vi "HV_drive.vi"(3 "Stop subVI Refnum":refnum<vi>, 4 "HV level Refnum":refnum<vi>, 5 "HV parameters":T1={"Final value"=-1000, "Number of steps"=10, "Time/step"=500, "Output Off Behavior"=0, "VISA resource name"="GPIB0::25::INSTR"} {"Output Off Behavior" items=["Normal", "High Impedance", "Zero", "Guard"]; "Time/step" min=100 max=2000 step=100; "Final value" min=-1100 max=0 step=10; "Number of steps" min=10 max=20 step=10}) -> (0 "error out":errorcluster, 2 "HV level (last value)":dbl(slide) scale=0.0..-1000.0)   [LabVIEW 2015, in "VIPM2.lvlib"]
uses:
  VIPM2.lvlib
  dr_Keithley 24XX/Keithley 24XX.lvlib
panel:
  # "Driver for the High Voltage Power Supply"
  # "Executa rampa de pujada o rampa de baixada"
  # "V"
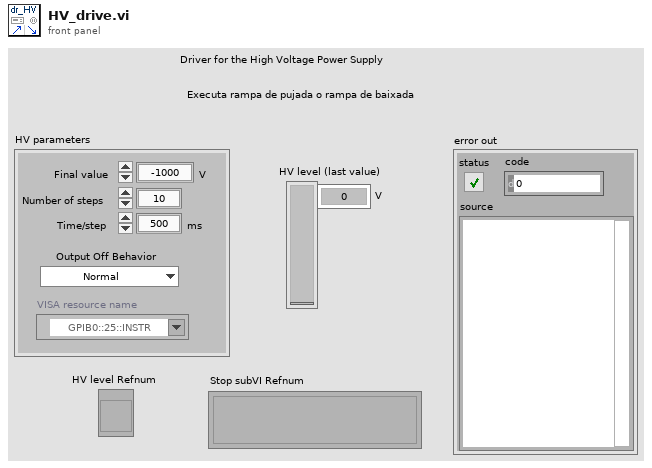
[diagram p1: front panel]
types:
  T1 = cluster{"Final value":i16, "Number of steps":u8, "Time/step":u16, "Output Off Behavior":u16, "VISA resource name":refnum<visa-resource-name>}
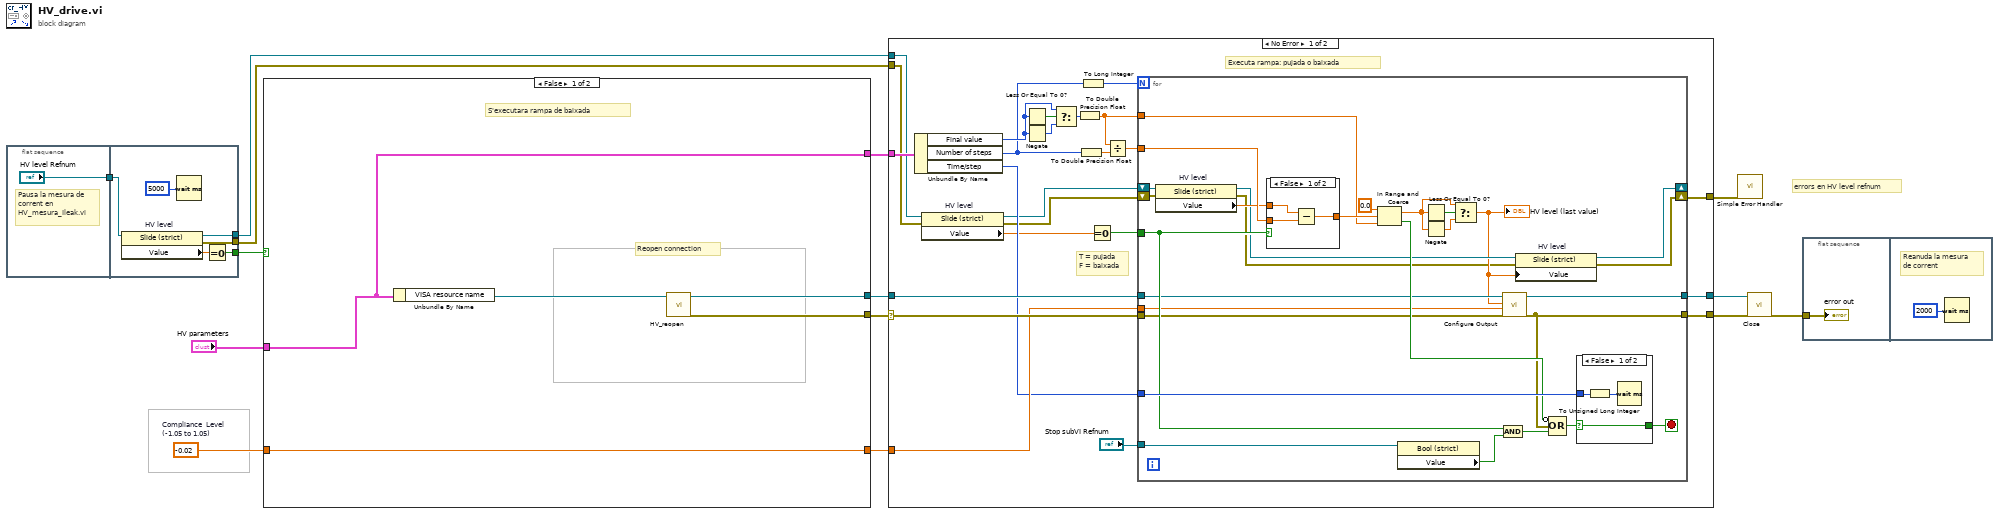
[diagram p0: block diagram]
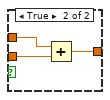
[diagram p3: hidden frame]
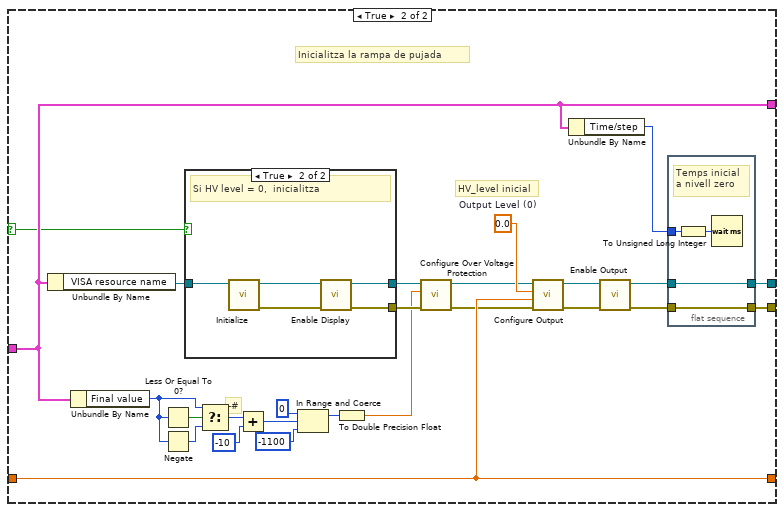
[diagram p5: hidden frame]
diagram:
  w12 = -0.02  # Compliance  Level (-1.05 to 1.05)
  # "errors en HV level refnum"
  n1 = flat-sequence {
    tunnel: ["HV level Refnum"] -> w7
    tunnel: [w21] -> w13
    tunnel: w7 -> [w19]
    tunnel: [w17] -> w6
    tunnel: [w16] -> w5
    frame #0 {
      # "Pausa la mesura de\ncorrent en\nHV_mesura_Ileak.vi"
    }
    frame #1 {
      n2 = property on="HV level" class="Slide (strict)"(reference=w19) -> (reference out=w17:refnum<vi>, error out=w16:errorcluster, "Value"=w18:dbl)  [unwired: 1 in]
      n3 = Wait (ms)(milliseconds to wait=u32 5000) -> ()  [unwired: 1 out]
      n4 = Equal To 0?(x=w18) -> (x = 0?=w21:bool)
    }
  }
  n5 = case shown="False" w13 {
    selector: w13 -> [_ w27]
    tunnel: "HV parameters" -> [w25 w40]
    tunnel: w12 -> [w26 w34]
    tunnel: [w24 w41] -> w9
    tunnel: [w23 w42] -> w10
    tunnel: [w26 w34] -> w8
    tunnel: [w25 w40] -> w11
    frame False {
      # "Reopen connection"
      # "S'executara rampa de baixada"
      n6 = Unbundle By Name(w25) -> ("VISA resource name"=w22:refnum<visa-resource-name>)
      n7 = call "HV_reopen.vi"("VISA resource name"=w22) -> ("error out"=w23:errorcluster, "VISA resource name out"=w24:refnum<visa-resource-name>)  [unwired: 9 in]
    }
    frame True {
      w33 = 0.0  # Output Level (0)
      # "HV_level inicial"
      # "Inicialitza la rampa de pujada"
      # "-#"
      n8 = Unbundle By Name(w40) -> ("VISA resource name"=w52:refnum<visa-resource-name>)
      n9 = Unbundle By Name(w40) -> ("Final value"=w50:i16)
      n10 = Less Or Equal To 0?(x=w50) -> (x <= 0?=w51:bool)
      n11 = Negate(x=w50) -> (-x=w49:i16)
      n12 = case shown="True" w27 {
        tunnel: [w53 w58] -> w29
        tunnel: [_ w57] -> w30
        tunnel: w52 -> [w53 w54]
        frame False {
        }
        frame True {
          # "Si HV level = 0,  inicialitza"
          n13 = call "Initialize.vi"("VISA resource name"=w54) -> ("error out"=w56:errorcluster, "VISA resource name out"=w55:refnum<visa-resource-name>)  [unwired: 9 in]
          n14 = call "Enable Display.vi"("error in (no error)"=w56, "VISA resource name"=w55) -> ("error out"=w57:errorcluster, "VISA resource name out"=w58:refnum<visa-resource-name>)  [unwired: 8 in]
        }
      }
      n15 = Select(t=w50, s=w51, f=w49) -> (s? t:f=w48:i16)
      n16 = Add(x=w48, y=i16 -10) -> (x+y=w46:i16)
      n17 = In Range and Coerce(upper limit=i16 0, x=w46, lower limit=i16 -1100) -> (coerced(x)=w43:i16)  [unwired: 1 out]
      n18 = To Double Precision Float(number=w43) -> (double precision float=w28:dbl)
      n19 = call "Configure Over Voltage Protection.vi"("error in (no error)"=w30, "Voltage Limit (0.0 V)"=w28, "VISA resource name"=w29) -> ("error out"=w32:errorcluster, "VISA resource name out"=w31:refnum<visa-resource-name>)  [unwired: 7 in]
      n20 = call "Configure Output.vi"("error in (no error)"=w32, "Compliance  Level (0.1)"=w34, "Output Level (0)"=w33, "VISA resource name"=w31) -> ("error out"=w36:errorcluster, "VISA resource name out"=w35:refnum<visa-resource-name>)  [unwired: 6 in]
      n21 = Unbundle By Name(w40) -> ("Time/step"=w39:u16)
      n22 = call "Enable Output.vi"("error in (no error)"=w36, "VISA resource name"=w35) -> ("error out"=w38:errorcluster, "VISA resource name out"=w37:refnum<visa-resource-name>)  [unwired: 8 in]
      n23 = flat-sequence {
        tunnel: w38 -> [w62]
        tunnel: [w62] -> w42
        tunnel: w37 -> [w61]
        tunnel: [w61] -> w41
        tunnel: w39 -> [w60]
        frame #0 {
          # "Temps inicial\na nivell zero"
          n24 = To Unsigned Long Integer(number=w60) -> (unsigned 32bit integer=w59:u32)
          n25 = Wait (ms)(milliseconds to wait=w59) -> ()  [unwired: 1 out]
        }
      }
    }
  }
  n26 = case shown="No Error" w10 {
    selector: w10 -> [w84 w126]
    tunnel: w11 -> [w86 _]
    tunnel: w9 -> [w85 w127]
    tunnel: w8 -> [w83 _]
    tunnel: [w79 w127] -> w2
    tunnel: [w78 w126] -> w3
    tunnel: w6 -> [w69 _]
    tunnel: w5 -> [w65 w125]
    tunnel: [w64 w125] -> w4
    frame No Error {
      # "Executa rampa: pujada o baixada"
      # "T = pujada\nF = baixada"
      n27 = Unbundle By Name(w86) -> ("Final value"=w75:i16, "Number of steps"=w70:u8, "Time/step"=w80:u16)
      n28 = property on="HV level" class="Slide (strict)"(reference=w69, error in=w65) -> (reference out=w67:refnum<vi>, error out=w66:errorcluster, "Value"=w68:dbl)
      n29 = Less Or Equal To 0?(x=w75) -> (x <= 0?=w76:bool)
      n30 = Negate(x=w75) -> (-x=w77:i16)
      n31 = Select(t=w75, s=w76, f=w77) -> (s? t:f=w74:i16)
      n32 = To Double Precision Float(number=w74) -> (double precision float=w73:dbl)
      n33 = To Double Precision Float(number=w70) -> (double precision float=w72:dbl)
      n34 = To Long Integer(number=w70) -> (32bit integer=w71:i32)
      n35 = Equal To 0?(x=w68) -> (x = 0?=w81:bool)
      n36 = Divide(x=w73, y=w72) -> (x/y=w82:dbl)
      n37 = for {
        N: w71 -> [_]
        tunnel: w85 -> [w98]
        tunnel: w84 -> [w99]
        tunnel: w83 -> [w97]
        tunnel: w82 -> [w114]
        tunnel: w81 -> [w111]
        tunnel: [w100] -> w79
        tunnel: [w101] -> w78
        tunnel: w80 -> [w113]
        tunnel: w73 -> [w104]
        shift-right: [w92] -> _
        shift-left: w67 -> [w96]
        shift-right: [w89] -> w64
        shift-left: w66 -> [w90]
        tunnel: "Stop subVI Refnum" -> [w88]
        stop <- w102 stop-if-true
        n38 = property on="HV level" class="Slide (strict)"(reference=w96, error in=w90) -> (reference out=w94:refnum<vi>, error out=w91:errorcluster, "Value"=w95:dbl)
        n39 = case shown="False" w111 {
          tunnel: w114 -> [w121 w122]
          tunnel: [w120 w124] -> w110
          tunnel: w95 -> [w119 w123]
          frame False {
            n40 = Subtract(x=w119, y=w121) -> (x-y=w120:dbl)
          }
          frame True {
            n41 = Add(x=w123, y=w122) -> (x+y=w124:dbl)
          }
        }
        n42 = In Range and Coerce(upper limit=0.0, x=w110, lower limit=w104) -> (coerced(x)=w106:dbl, In Range?=w105:bool)
        n43 = property class="Bool (strict)"(reference=w88) -> ("Value"=w87:bool)  [unwired: 1 in, 2 out]
        n44 = Less Or Equal To 0?(x=w106) -> (x <= 0?=w107:bool)
        n45 = Negate(x=w106) -> (-x=w108:dbl)
        n46 = Select(t=w106, s=w107, f=w108) -> (s? t:f=w93:dbl)
        "HV level (last value)" <- w93
        n47 = And(x=w111, y=w87) -> (x .and. y?=w112:bool)
        n48 = call "Configure Output.vi"("error in (no error)"=w99, "Compliance  Level (0.1)"=w97, "Output Level (0)"=w93, "VISA resource name"=w98) -> ("error out"=w101:errorcluster, "VISA resource name out"=w100:refnum<visa-resource-name>)  [unwired: 6 in]
        n49 = property on="HV level" class="Slide (strict)"(reference=w94, error in=w91, "Value"=w93) -> (reference out=w92:refnum<vi>, error out=w89:errorcluster)
        n50 = Compound Arithmetic op=OR(invert w105, w101, w112) -> (w103:bool)
        n51 = case shown="False" w103 {
          selector: w103 -> [w117 w118]
          tunnel: w113 -> [w116 _]
          tunnel: [w117 w118] -> w102
          frame False {
            n52 = To Unsigned Long Integer(number=w116) -> (unsigned 32bit integer=w115:u32)
            n53 = Wait (ms)(milliseconds to wait=w115) -> ()  [unwired: 1 out]
          }
          frame True {
            # "per aturar\nno temps"
          }
        }
      }
    }
    frame Error {
    }
  }
  n54 = call <vilib>:"Simple Error Handler.vi"("error in (no error)"=w4) -> ()  [unwired: 4 in, 5 out]
  n55 = call "Close.vi"("error in (no error)"=w3, "VISA resource name"=w2) -> ("error out"=w1:errorcluster)  [unwired: 9 in]
  n56 = flat-sequence {
    tunnel: w1 -> [w128]
    frame #0 {
      "error out" <- w128
    }
    frame #1 {
      # "Reanuda la mesura\nde corrent"
      n57 = Wait (ms)(milliseconds to wait=u32 2000) -> ()  [unwired: 1 out]
    }
  }
